vi "ReadRowU16.vi"(8 "error in":errorcluster, 10 "Row":i32, 11 "Image Reference In":T1) -> (0 "error out":errorcluster, 2 "Pixel Row":u16[](array[numeric]), 3 "Image Reference Out":T1)   [LabVIEW 2020, in "OpenLvVision_Image.lvlib" / "DataAccess.lvlib"]
doc: "Returns the values of an pixel row"
uses:
  DataAccess.lvlib
  Management/TypeDef/Image.ctl
  <vilib>/Utility/error.llb/Error Cluster From Error Code.vi
  <vilib>/ErrorRing/Error Ring.xnode
  Management/Management.lvlib
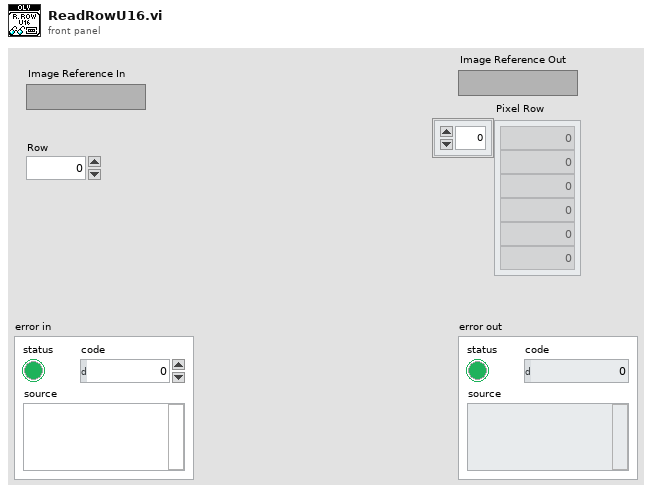
[diagram p1: front panel]
types:
  T1 = typedef "OpenLvVision_Image.lvlib/Management.lvlib/Image.ctl" = refnum<image>
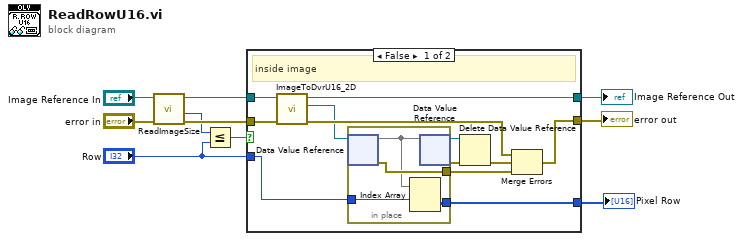
[diagram p0: block diagram]
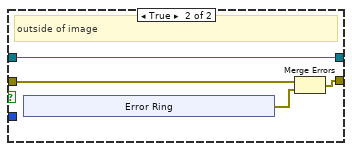
[diagram p2: hidden frame]
diagram:
  n1 = call "ReadImageSize.vi"("error in"="error in", "Image Reference In"="Image Reference In") -> ("error out"=w9:errorcluster, "Height"=w1:i32, "Image Reference Out"=w10:T1)  [unwired: 6 in, 1 out]
  n2 = Less Or Equal?(x=w1, y="Row") -> (x <= y?=w4:bool)
  n3 = case shown="False" w4 {
    tunnel: w10 -> [w22 w28]
    tunnel: w9 -> [w21 w30]
    tunnel: [w20 w28] -> w6
    tunnel: [w12 w27] -> w5
    tunnel: [w13 _] -> w2
    tunnel: "Row" -> [w11 _]
    frame False {
      # "inside image"
      n4 = call "ImageToDvrU16_2D.vi"("error in"=w21, "Image Reference In"=w22) -> ("error out"=w15:errorcluster, "EDVR 2D U16"=w14:refnum<data-value>, "Image Reference Out"=w20:T1)  [unwired: 6 in, 1 out]
      n5 = in-place {
        in-place-border: [w26] -> w18
        in-place-border: [w24] -> w13
        in-place-border: w11 -> [w23]
        n6 = in-place-dvr #1(w14) -> (w25:u16[][], w26:errorcluster)
        n7 = Index Array(array=w25, index (row)=w23) -> (element=w24:u16[])  [unwired: 1 in]
        n8 = in-place-dvr #1(w25) -> (w16:refnum<data-value>, w17:errorcluster)
      }
      n9 = Delete Data Value Reference(data value reference=w16, error in=w17) -> (error out=w19:errorcluster)  [unwired: 1 out]
      n10 = Merge Errors(w15, w19, w18) -> (w12:errorcluster)
    }
    frame True {
      # "outside of image"
      n11 = xnode "Error Ring"() -> ("error out"=w29:errorcluster)
      n12 = Merge Errors(w30, w29) -> (w27:errorcluster)
    }
  }
  "error out" <- w5
  "Image Reference Out" <- w6
  "Pixel Row" <- w2
